vi "CreateQueue.vi"(8 "error in (no error)":errorcluster, 11 "QueueName":string) -> (0 "error out":errorcluster, 3 "QueueOUT":refnum<queue>)   [LabVIEW 2018]
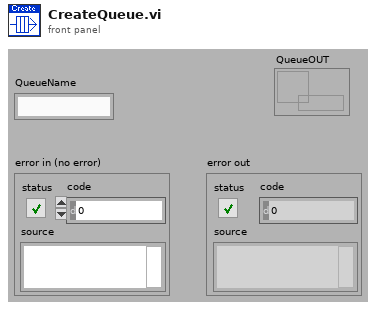
[diagram p1: front panel]
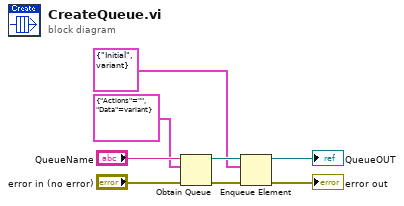
[diagram p0: block diagram]
diagram:
  n1 = Obtain Queue(name (unnamed)="QueueName", element data type=cluster{"Actions":string, "Data":variant} {"Actions"="", "Data"=variant}, error in (no error)="error in (no error)") -> (queue out=w5:refnum<queue>, error out=w6:errorcluster)  [unwired: 2 in, 1 out]
  n2 = Enqueue Element(queue=w5, element=cluster{"Actions":string, "Data":variant} {"Actions"="Initial", "Data"=variant} ("元素"), error in (no error)=w6) -> (queue out=→"QueueOUT":refnum<queue>, error out=→"error out":errorcluster)  [unwired: 2 out]
